vi "Insert BCD Parameter.vi"(8 "Signed?":bool, 9 "Number of Bits":T1=1 min=1 max=32, 10 "Start Bit":T2, 11 "BCD Value":dbl=25786.0) -> (1 "BCD Mask":bool[](array[boolean]), 3 "U32":u32)   [LabVIEW 2020]
uses:
  Shared/Controls and Global/Start Bit.ctl
  Shared/Controls and Global/Number of Bits.ctl
  Shared/Ballard Arinc-429 Shared.lvlib
panel:
  out "Char 1":i32
  out "Char 2":i32
  out "Char 3":i32
  out "Char 4":i32
  out "Char 5":i32
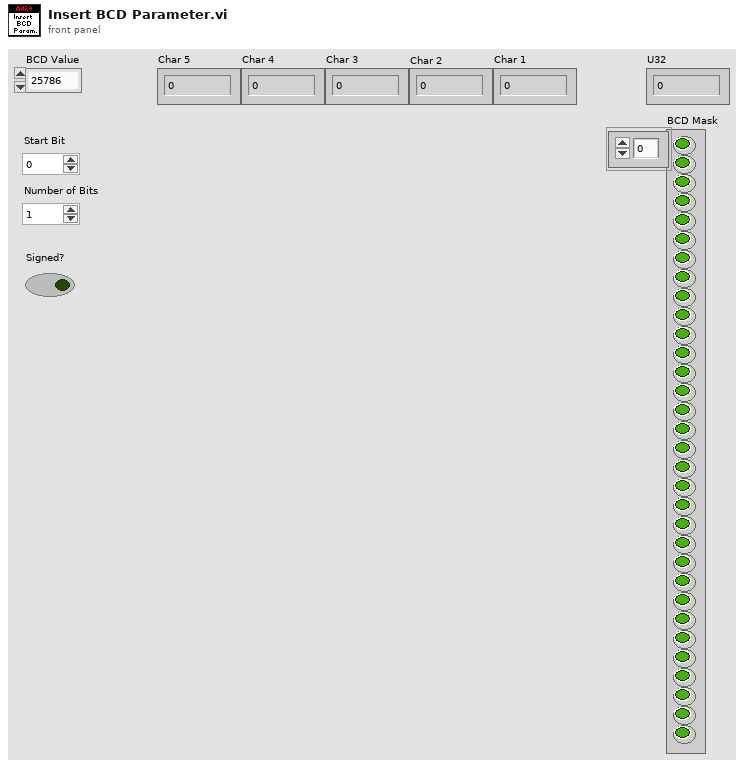
[diagram p1: front panel]
types:
  T1 = typedef "Ballard Arinc-429 Shared.lvlib/Number of Bits.ctl" = i32
  T2 = typedef "Ballard Arinc-429 Shared.lvlib/Start Bit.ctl" = i32
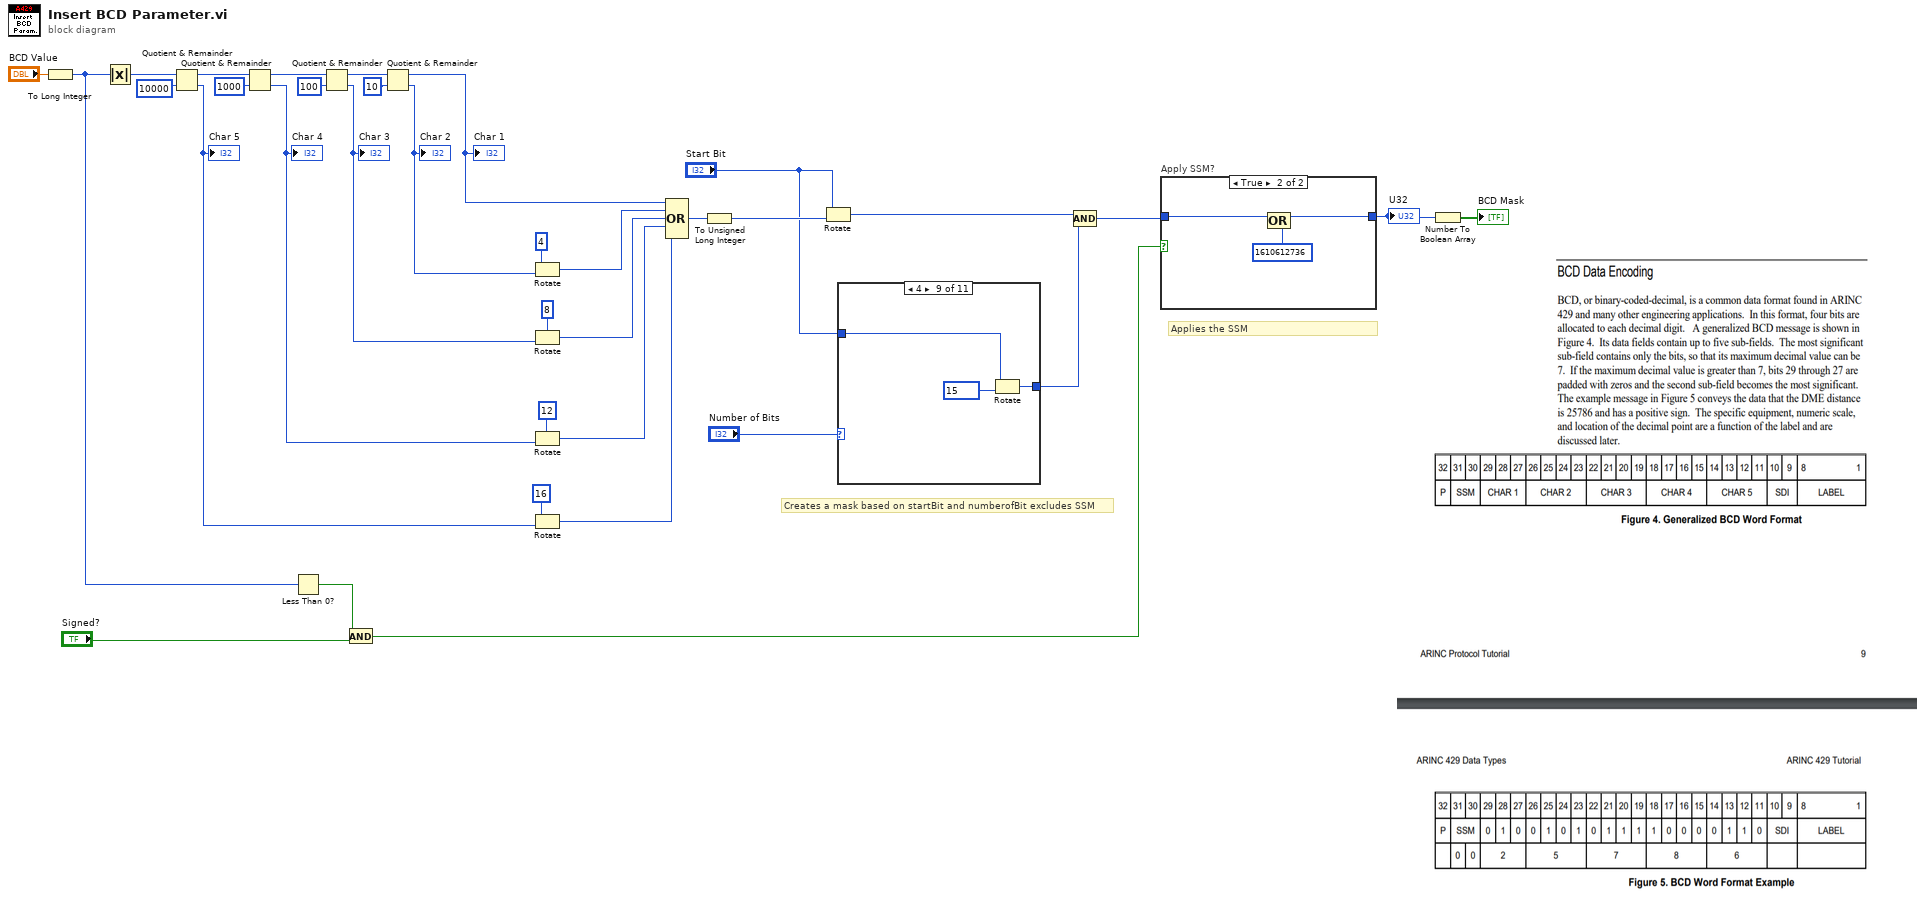
[diagram p0: block diagram]
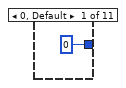
[diagram p2: hidden frame]
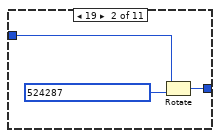
[diagram p3: hidden frame]
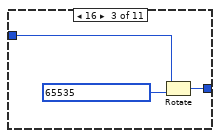
[diagram p4: hidden frame]
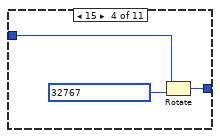
[diagram p5: hidden frame]
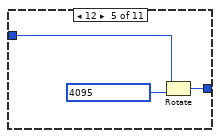
[diagram p6: hidden frame]
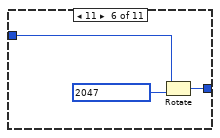
[diagram p7: hidden frame]
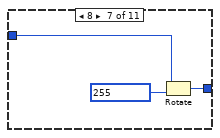
[diagram p8: hidden frame]
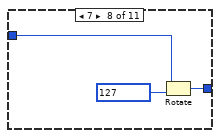
[diagram p9: hidden frame]
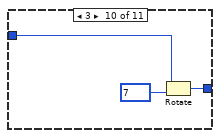
[diagram p10: hidden frame]
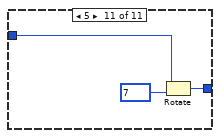
[diagram p11: hidden frame]
diagram:
  # "Applies the SSM"
  # "Creates a mask based on startBit and numberofBit excludes SSM"
  n1 = To Long Integer(number="BCD Value") -> (32bit integer=w3:i32)
  n2 = Absolute Value(x=w3) -> (abs(x)=w11:i32)
  n3 = Quotient & Remainder(x=w11, y=10000) -> (x-y*floor(x/y)=w34:i32, floor(x/y)=w20:i32)
  "Char 5" <- w20
  n4 = Quotient & Remainder(x=w34, y=1000) -> (x-y*floor(x/y)=w32:i32, floor(x/y)=w23:i32)
  "Char 4" <- w23
  n5 = Less Than 0?(x=w3) -> (x < 0?=w13:bool)
  n6 = Quotient & Remainder(x=w32, y=100) -> (x-y*floor(x/y)=w29:i32, floor(x/y)=w26:i32)
  "Char 3" <- w26
  n7 = And(x=w13, y="Signed?") -> (x .and. y?=w12:bool)
  n8 = Quotient & Remainder(x=w29, y=10) -> (x-y*floor(x/y)=w16:i32, floor(x/y)=w28:i32)
  "Char 2" <- w28
  "Char 1" <- w16
  n9 = Rotate(1:w28, 2:i16 4 ("y")) -> (0:w15:i32)
  n10 = Rotate(1:w26, 2:i16 8 ("y")) -> (0:w22:i32)
  n11 = Rotate(1:w23, 2:i16 12 ("y")) -> (0:w21:i32)
  n12 = Rotate(1:w20, 2:i16 16 ("y")) -> (0:w18:i32)
  n13 = Compound Arithmetic op=OR(w16, w15, w22, w21, w18) -> (w10:i32)
  n14 = To Unsigned Long Integer(number=w10) -> (unsigned 32bit integer=w7:u32)
  n15 = Rotate(1:w7, 2:"Start Bit") -> (0:w6:u32)
  n16 = case shown="4" "Number of Bits" {
    tunnel: "Start Bit" -> [_ w37 w40 w43 w46 w49 w52 w55 w58 w61 w64]
    tunnel: [u32 0 w38 w41 w44 w47 w50 w53 w56 w59 w62 w65] -> w8
    frame 0, Default {
    }
    frame 19 {
      n17 = Rotate(1:u32 524287 ("y"), 2:w37) -> (0:w38:u32)
    }
    frame 16 {
      n18 = Rotate(1:u32 65535 ("y"), 2:w40) -> (0:w41:u32)
    }
    frame 15 {
      n19 = Rotate(1:u32 32767 ("y"), 2:w43) -> (0:w44:u32)
    }
    frame 12 {
      n20 = Rotate(1:u32 4095 ("y"), 2:w46) -> (0:w47:u32)
    }
    frame 11 {
      n21 = Rotate(1:u32 2047 ("y"), 2:w49) -> (0:w50:u32)
    }
    frame 8 {
      n22 = Rotate(1:u32 255 ("y"), 2:w52) -> (0:w53:u32)
    }
    frame 7 {
      n23 = Rotate(1:u32 127 ("y"), 2:w55) -> (0:w56:u32)
    }
    frame 4 {
      n24 = Rotate(1:u32 15 ("y"), 2:w58) -> (0:w59:u32)
    }
    frame 3 {
      n25 = Rotate(1:u32 7 ("y"), 2:w61) -> (0:w62:u32)
    }
    frame 5 {
      n26 = Rotate(1:u32 7 ("y"), 2:w64) -> (0:w65:u32)
    }
  }
  n27 = Compound Arithmetic op=AND(w6, w8) -> (w9:u32)
  n28 = case "Apply SSM?" shown="True" w12 {
    tunnel: w9 -> [w67 w70]
    tunnel: [w67 w69] -> w5
    frame False {
    }
    frame True {
      n29 = Compound Arithmetic op=OR(w70, u32 1610612736 ("number 2")) -> (w69:u32)
    }
  }
  "U32" <- w5
  n30 = Number To Boolean Array(number=w5) -> (Boolean array=→"BCD Mask":bool[])
